vi "Read Vendor Name.vi"(8 "error in (no error)":errorcluster, 11 "Asset in":refnum<class "Asset.lvclass">) -> (0 "error out":errorcluster, 2 "vendor name":string, 3 "Asset out":refnum<class "Asset.lvclass">)   [LabVIEW 2019, in "Asset.lvclass"]
uses:
  Asset.lvclass
  Asset.lvclass/Asset.ctl
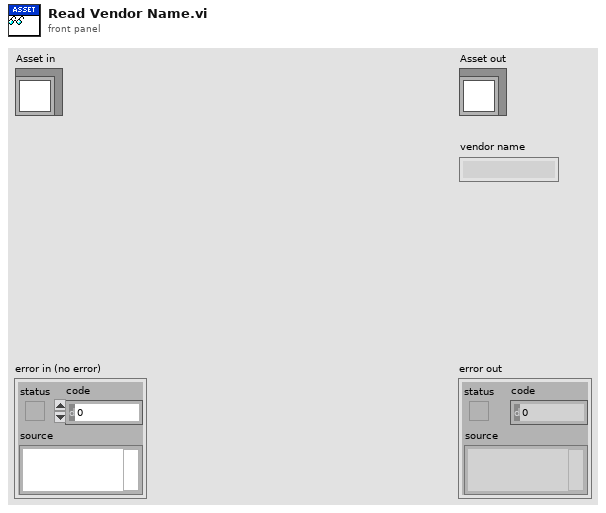
[diagram p1: front panel]
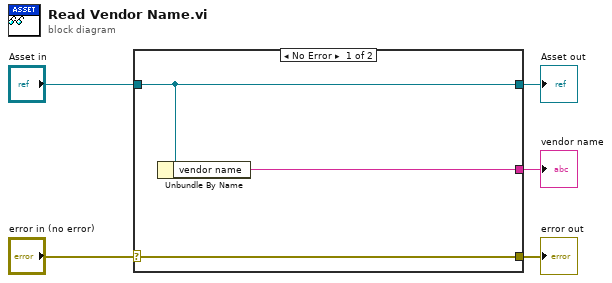
[diagram p0: block diagram]
diagram:
  n1 = case shown="No Error" "error in (no error)" {
    selector: "error in (no error)" -> [w8 w9]
    tunnel: [w8 w9] -> w4
    tunnel: [w7 w10] -> w2
    tunnel: "Asset in" -> [w7 w10]
    tunnel: [w6 _] -> w1
    frame No Error {
      n2 = Unbundle By Name(w7) -> ("vendor name"=w6:string)
    }
    frame Error {
    }
  }
  "error out" <- w4
  "Asset out" <- w2
  "vendor name" <- w1
